vi "PS FPGA Filter Read Coefficients.vi"(11 "offset":u8) -> (2 "a coeffs":fxp<+/-,20,2>[](array[numeric]), 3 "b coeffs":fxp<+/-,20,2>[](array[numeric]))   [LabVIEW 2011]
uses:
  <vilib>/rvi/Memory/Memory_Emulation/niFpgaMemoryEmulationValidateCache.vi
  <vilib>/rvi/DataTransferAndStorage/Container/Common/niFpgaContainerGetUniqueNameForEmu.vi
  <vilib>/rvi/Memory/Memory_Emulation/nirvimemoryEmulationManagerCache_InsertValue.vi
  <vilib>/Utility/error.llb/Clear Errors.vi
  <vilib>/rvi/Memory/Memory_Emulation/nirvimemoryEmulationManagerCache_GetValue.vi
  <vilib>/rvi/DataTransferAndStorage/Container/XNode/niFpgaContainer.xnode
  <vilib>/rvi/Memory/Memory_Emulation/nirvimemoryEmulation.vi
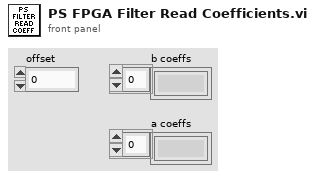
[diagram p1: front panel]
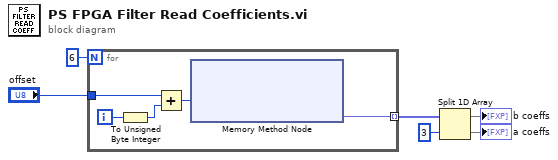
[diagram p0: block diagram]
diagram:
  n1 = for {
    N: 6 -> [_]
    tunnel: [w8] -> w3 mode=indexing
    tunnel: "offset" -> [w7]
    i -> [w11]
    n2 = To Unsigned Byte Integer(number=w11) -> (unsigned 8bit integer=w10:u8)
    n3 = Add(x=w7, y=w10) -> (x+y=w9:u8)
    n4 = xnode ("Memory Method Node")("Address"=w9) -> ("Data"=w8:fxp<+/-,20,2>)  [unwired: 1 in, 1 out]
  }
  n5 = Split 1D Array(array=w3, index=3) -> (first subarray=→"b coeffs":fxp<+/-,20,2>[], second subarray=→"a coeffs":fxp<+/-,20,2>[])
